vi "subtract.vi"(7 "Request in":refnum<class "Request.lvclass">, 8 "error in (no error)":errorcluster, 10 "params":variant, 11 "Server in":refnum<class "JSONRPC Server.lvclass">) -> (0 "error out":errorcluster, 3 "JSONRPC Server out":refnum<class "JSONRPC Server.lvclass">)   [LabVIEW 2016]
uses:
  Classes/Request/Request.lvclass
  Classes/Server/JSONRPC Server.lvclass
  <vilib>/rajsite/i3-json/JSON Parsing/Get Array Value at Index Files/Get Array Value at Index - Numeric.vi
  <vilib>/rajsite/i3-json/JSON Generation/Create Value Files/Create Value - Numeric.vi
  Classes/Server/Add Response (Result from Request).vi
  Classes/Server/Add Response (Invalid Params from Request).vi
  <vilib>/rajsite/i3-json/i3-json.lvlib
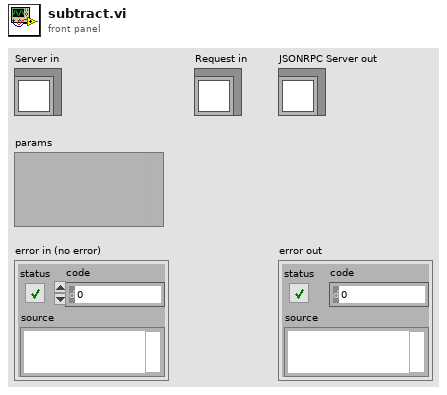
[diagram p1: front panel]
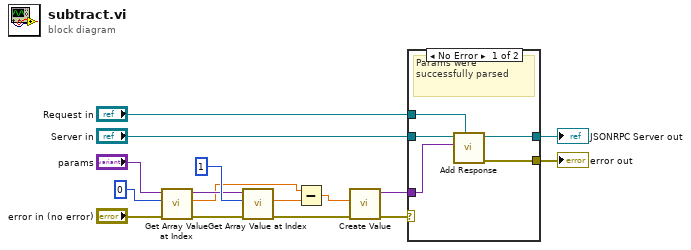
[diagram p0: block diagram]
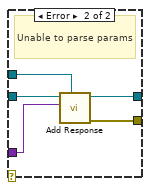
[diagram p2: hidden frame]
diagram:
  n1 = call-poly <vilib>:"Get Array Value at Index.vi"("error in (no error)"="error in (no error)", "Index"=0, "JSON Tree In (JSON Array)"="params") -> ("error out"=w7:errorcluster, "Double Value"=w2:dbl, "JSON Tree Out Passthrough"=w5:variant)  [unwired: 5 in, 1 out]
  n2 = call-poly <vilib>:"Get Array Value at Index.vi"("error in (no error)"=w7, "Index"=1, "JSON Tree In (JSON Array)"=w5) -> ("error out"=w8:errorcluster, "Double Value"=w3:dbl)  [unwired: 5 in, 2 out]
  n3 = Subtract(x=w2, y=w3) -> (x-y=w1:dbl)
  n4 = call-poly <vilib>:"Create Value.vi"("error in (no error)"=w8, "Numeric"=w1) -> ("error out"=w16:errorcluster, "JSON Tree"=w13:variant)  [unwired: 8 in]
  n5 = case shown="No Error" w16 {
    tunnel: "Server in" -> [w21 w26]
    tunnel: [w20 w25] -> w12
    tunnel: w13 -> [w19 w24]
    tunnel: [w18 w23] -> w14
    tunnel: "Request in" -> [w17 w22]
    frame No Error {
      # "Params were successfully parsed"
      n6 = call-poly "Add Response.vi"("Request"=w17, "Response JSON Tree In"=w19, "Server in"=w21) -> ("error out"=w18:errorcluster, "Server out"=w20:refnum<class "JSONRPC Server.lvclass">)  [unwired: 6 in, 1 out]
    }
    frame Error {
      # "Unable to parse params"
      n7 = call-poly "Add Response.vi"("Request"=w22, "data"=w24, "Server in"=w26) -> ("error out"=w23:errorcluster, "Server out"=w25:refnum<class "JSONRPC Server.lvclass">)  [unwired: 6 in, 1 out]
    }
  }
  "error out" <- w14
  "JSONRPC Server out" <- w12
